vi "GetPPIXImg.vi"(8 "Background":dbl, 9 "dy":dbl, 10 "Origin":cluster{"X":sgl, "Y":sgl, "Z":sgl}, 11 "3D Profile in":cluster{"x(mm)":dbl, "y(mm)":dbl, "z(mm)":dbl}[](array[cluster])) -> (0 "Z":dbl[](array[numeric]), 1 "Y":dbl[](array[numeric]), 2 "X":dbl[](array[numeric]), 3 "3D Profile":cluster{"x(mm)":dbl, "y(mm)":dbl, "z(mm)":dbl}[](array[cluster]))   [LabVIEW 2024]
panel:
  out "Z":dbl[](graph)
  out "Y":dbl[](graph)
  out "X":dbl[](graph)
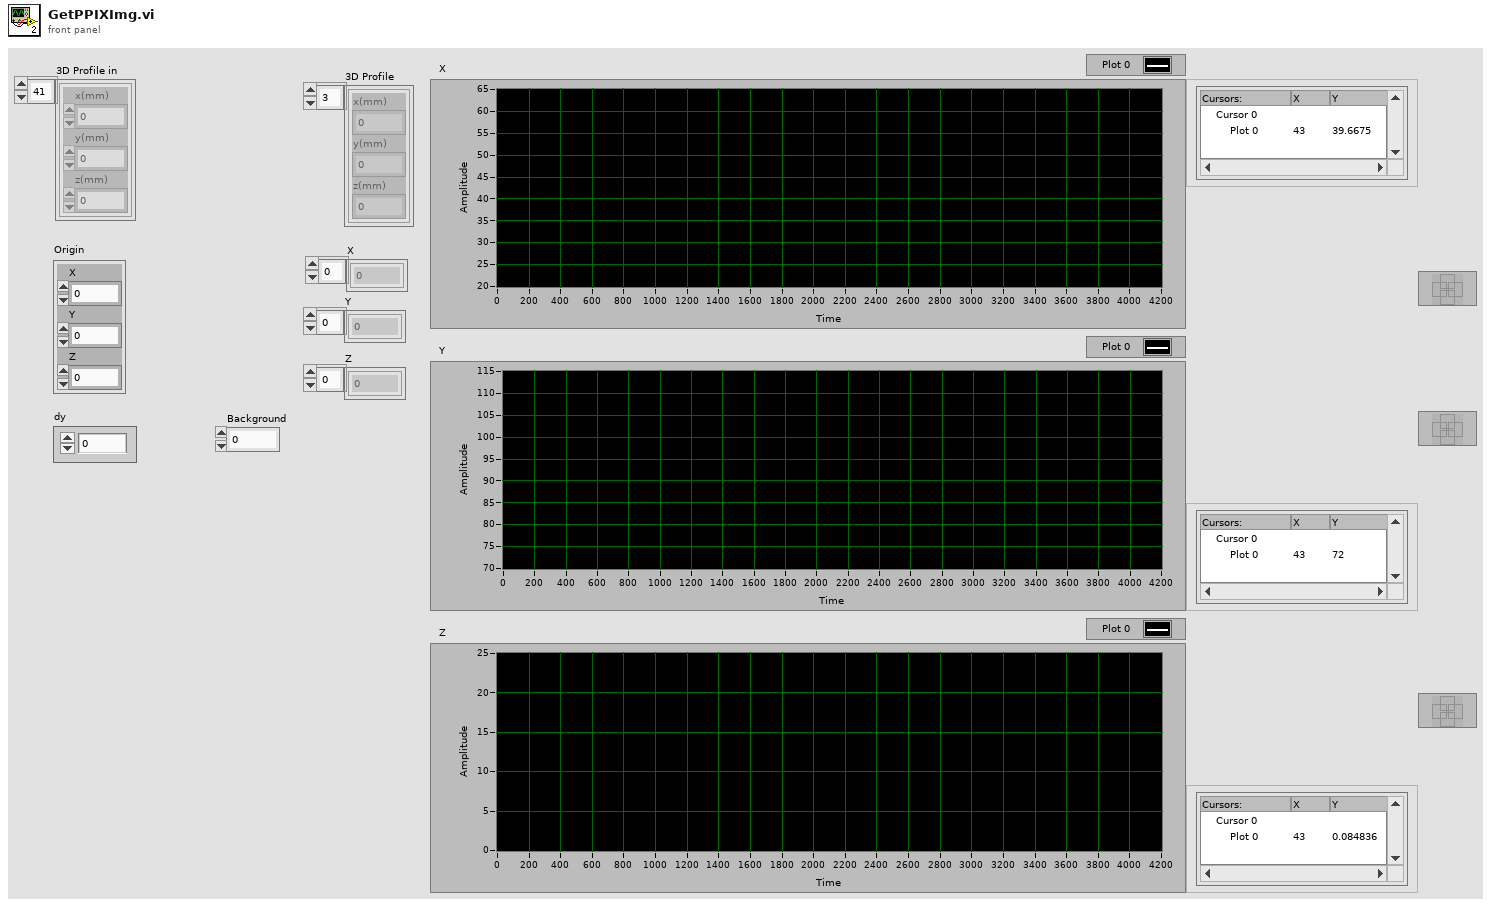
[diagram p1: front panel]
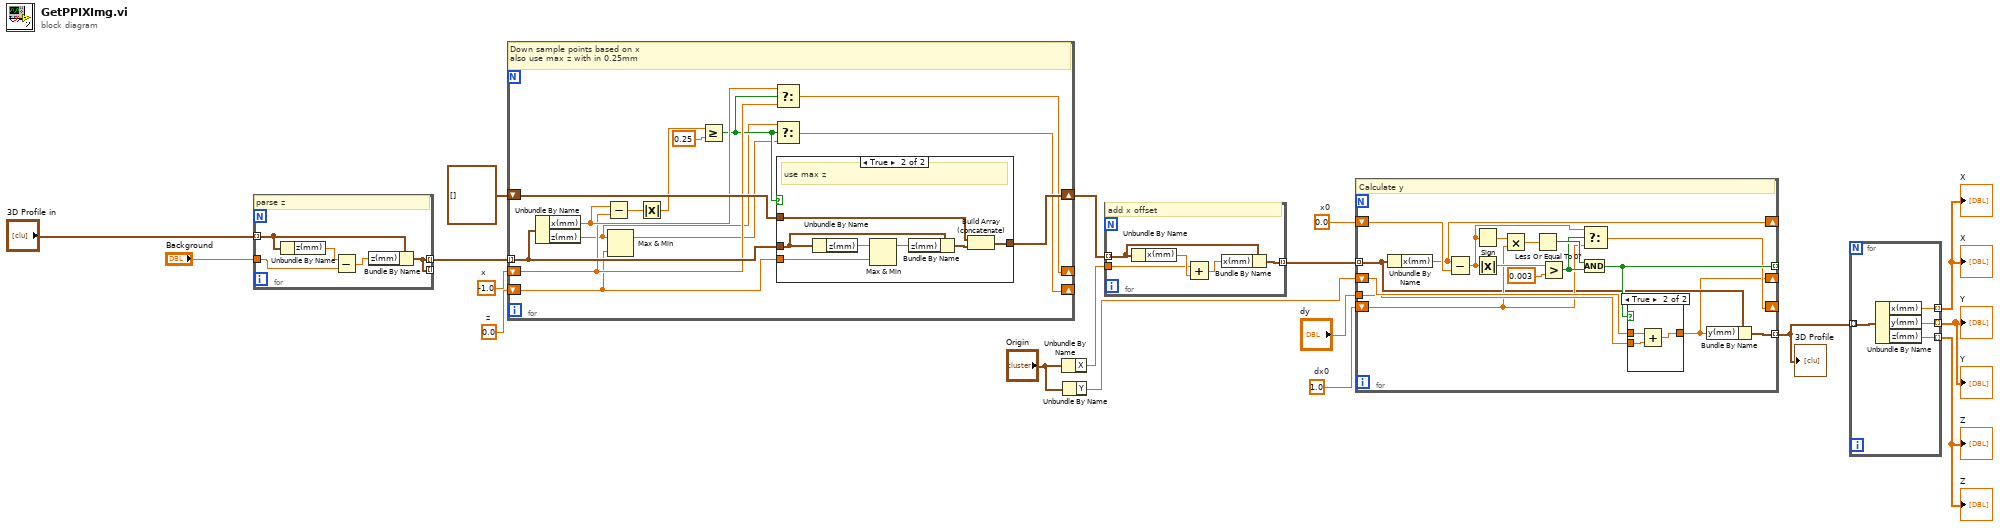
[diagram p0: block diagram]
diagram:
  w6 = 0.0  # z
  w15 = 1.0  # dx0
  w16 = 0.0  # x0
  w17 = -1.0  # x
  n1 = for {
    tunnel: "Background" -> [w19]
    tunnel: "3D Profile in" -> [w23] mode=indexing
    tunnel: [w21] -> _ mode=indexing
    tunnel: [w21] -> w7 mode=indexing
    # "parse z"
    n2 = Unbundle By Name(w23) -> ("z(mm)"=w20:dbl)
    n3 = Subtract(x=w20, y=w19) -> (x-y=w22:dbl)
    n4 = Bundle By Name(cluster=w23, "z(mm)"=w22) -> (w21:cluster{"x(mm)":dbl, "y(mm)":dbl, "z(mm)":dbl})
  }
  n5 = for {
    tunnel: w7 -> [w34] mode=indexing
    shift-right: [w30] -> _
    shift-left: w17 -> [w31]
    shift-right: [w33] -> w10
    shift-left: cluster{"x(mm)":dbl, "y(mm)":dbl, "z(mm)":dbl}[] [] -> [w35]
    shift-right: [w27] -> _
    shift-left: w6 -> [w24]
    # "Down sample points based on x\nalso use max z with in 0.25mm"
    n6 = Unbundle By Name(w34) -> ("x(mm)"=w32:dbl, "z(mm)"=w26:dbl)
    n7 = Subtract(x=w32, y=w31) -> (x-y=w37:dbl)
    n8 = Max & Min(x=w26, y=w24) -> (max(x,y)=w25:dbl)  [unwired: 1 out]
    n9 = Absolute Value(x=w37) -> (abs(x)=w29:dbl)
    n10 = Greater Or Equal?(x=w29, y=0.25) -> (x >= y?=w28:bool)
    n11 = Select(t=w32, s=w28, f=w31) -> (s? t:f=w30:dbl)
    n12 = Select(t=w26, s=w28, f=w25) -> (s? t:f=w27:dbl)
    n13 = case shown="True" w28 {
      tunnel: w35 -> [w38 w45]
      tunnel: w34 -> [_ w41]
      tunnel: [w38 w44] -> w33
      tunnel: w24 -> [_ w42]
      frame False {
      }
      frame True {
        # "use max z"
        n14 = Unbundle By Name(w41) -> ("z(mm)"=w43:dbl)
        n15 = Max & Min(x=w43, y=w42) -> (max(x,y)=w40:dbl)  [unwired: 1 out]
        n16 = Bundle By Name(cluster=w41, "z(mm)"=w40) -> (w39:cluster{"x(mm)":dbl, "y(mm)":dbl, "z(mm)":dbl})
        n17 = Build Array (concatenate)(w45, w39) -> (w44:cluster{"x(mm)":dbl, "y(mm)":dbl, "z(mm)":dbl}[])
      }
    }
  }
  n18 = Unbundle By Name("Origin") -> ("X"=w11:sgl)
  n19 = Unbundle By Name("Origin") -> ("Y"=w13:sgl)
  n20 = for {
    tunnel: w10 -> [w48] mode=indexing
    tunnel: w11 -> [w49]
    tunnel: [w46] -> w9 mode=indexing
    # "add x offset"
    n21 = Unbundle By Name(w48) -> ("x(mm)"=w50:dbl)
    n22 = Add(x=w49, y=w50) -> (x+y=w47:dbl)
    n23 = Bundle By Name(cluster=w48, "x(mm)"=w47) -> (w46:cluster{"x(mm)":dbl, "y(mm)":dbl, "z(mm)":dbl})
  }
  n24 = for {
    tunnel: w9 -> [w54] mode=indexing
    shift-right: [w51] -> _
    shift-left: w16 -> [w67]
    shift-right: [w56] -> _
    shift-left: w15 -> [w55]
    shift-right: [w53] -> _
    shift-left: w13 -> [w65]
    tunnel: "dy" -> [w64]
    tunnel: [w52] -> w5 mode=indexing
    tunnel: [w59] -> _ mode=indexing
    # "Calculate y"
    n25 = Unbundle By Name(w54) -> ("x(mm)"=w51:dbl)
    n26 = Subtract(x=w51, y=w67) -> (x-y=w57:dbl)
    n27 = Sign(1:w57) -> (0:w63:dbl)
    n28 = Absolute Value(x=w57) -> (abs(x)=w62:dbl)
    n29 = Multiply(x=w63, y=w55) -> (x*y=w66:dbl)
    n30 = Less Or Equal To 0?(x=w66) -> (x <= 0?=w60:bool)
    n31 = Greater?(x=w62, y=0.003) -> (0:w58:bool)
    n32 = And(x=w60, y=w58) -> (x .and. y?=w59:bool)
    n33 = Select(t=w57, s=w58, f=w55) -> (s? t:f=w56:dbl)
    n34 = case shown="True" w59 {
      tunnel: w65 -> [w68 w70]
      tunnel: [w68 w71] -> w53
      tunnel: w64 -> [_ w69]
      frame False {
      }
      frame True {
        n35 = Add(x=w70, y=w69) -> (x+y=w71:dbl)
      }
    }
    n36 = Bundle By Name(cluster=w54, "y(mm)"=w53) -> (w52:cluster{"x(mm)":dbl, "y(mm)":dbl, "z(mm)":dbl})
  }
  "3D Profile" <- w5
  n37 = for {
    tunnel: w5 -> [w75] mode=indexing
    tunnel: [w74] -> w3 mode=indexing
    tunnel: [w73] -> w2 mode=indexing
    tunnel: [w72] -> w4 mode=indexing
    n38 = Unbundle By Name(w75) -> ("x(mm)"=w74:dbl, "y(mm)"=w73:dbl, "z(mm)"=w72:dbl)
  }
  "Y" <- w2
  "X" <- w3
  "X" <- w3
  "Y" <- w2
  "Z" <- w4
  "Z" <- w4
